vi "AutomaticSend.vi"() -> ()   [LabVIEW 2020, in "zlgcan.lvlib"]
uses:
  zlgcan.lvlib
panel:
  in  "Auto CAN Data":T1={"Send ID"=18, "CANFD_SpeedUp"=0, "agreement"=0, "frame type"=0, "can_index_handle"=0, "milliseconds to wait"=1000, "Data"="11 22 33 44 55 66 77 88"} {"Send ID" format="0x%08x"}
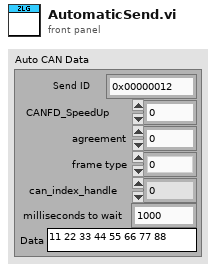
[diagram p1: front panel]
types:
  T1 = cluster{"Send ID":u32, "CANFD_SpeedUp":u32, "agreement":u32, "frame type":u32, "can_index_handle":u32, "milliseconds to wait":u32, "Data":string}
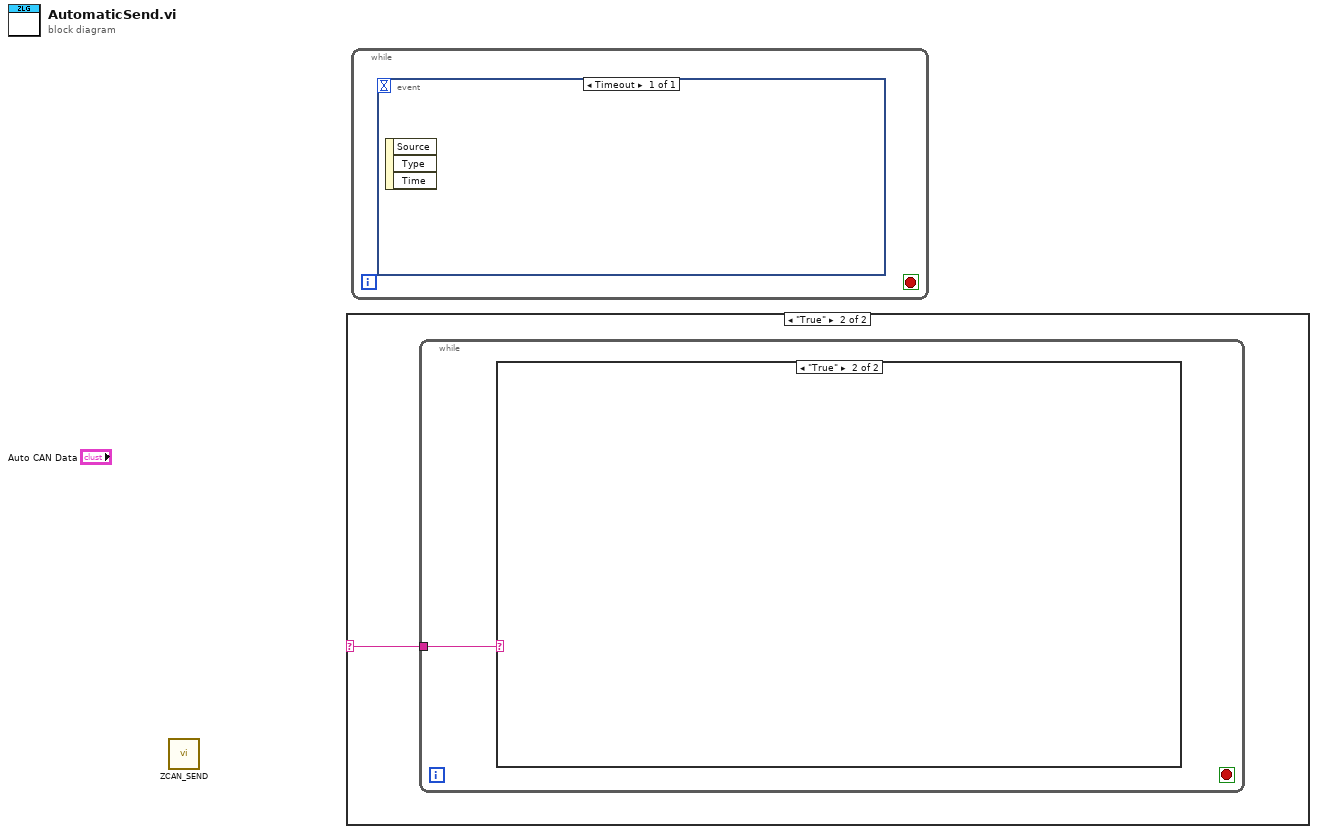
[diagram p0: block diagram]
diagram:
  n1 = call "ZCAN_SEND.vi"() -> ()  [unwired: 10 in, 2 out]
  n2 = case shown="\"True\"" {
    selector: _ -> [_ w1]
    frame "False", Default {
    }
    frame "True" {
      n3 = while {
        tunnel: w1 -> [w2]
        stop <- _ stop-if-true
        n4 = case shown="\"True\"" w2 {
          frame "False", Default {
          }
          frame "True" {
          }
        }
      }
    }
  }
  n5 = while {
    stop <- _ stop-if-true
    n6 = event shown="[0] Timeout" {
      selector: _ -> [_]
      dyn-events: _ -> [_]
      timeout: _ -> [_]
      event Timeout {
        n7 = event-data() -> ()  [unwired: 1 in, 3 out]
      }
    }
  }
